vi "Normalize Results.vi"(8 "Sorted Data":dbl[][](array[numeric]), 11 "Image in":T2) -> (3 "Results":T1(array[cluster]) {"Score" format="%#_3g"; "Pixels"."Rectangle"."Numeric 5" format="%#_3g"; "Pixels"."Rectangle"."Numeric 3" format="%#_3g"; "Pixels"."Rectangle"."Numeric 2" format="%#_3g"; "Pixels"."Rectangle"."Numeric" format="%#_3g"; "Normalized"."Rectangle"."Numeric 5" format="%#_2g"; "Normalized"."Rectangle"."Numeric 3" format="%#_2g"; "Normalized"."Rectangle"."Numeric 2" format="%#_2g"; "Normalized"."Rectangle"."Numeric" format="%#_2g"; "Normalized"."Center"."?" format="%#_3g"; "Normalized"."Center"."?" format="%#_3g"; "Distance (ft)" format="%#_3g"})   [LabVIEW 2016]
uses:
  <vilib>/vision/Image Controls.llb/IMAQ Image.ctl
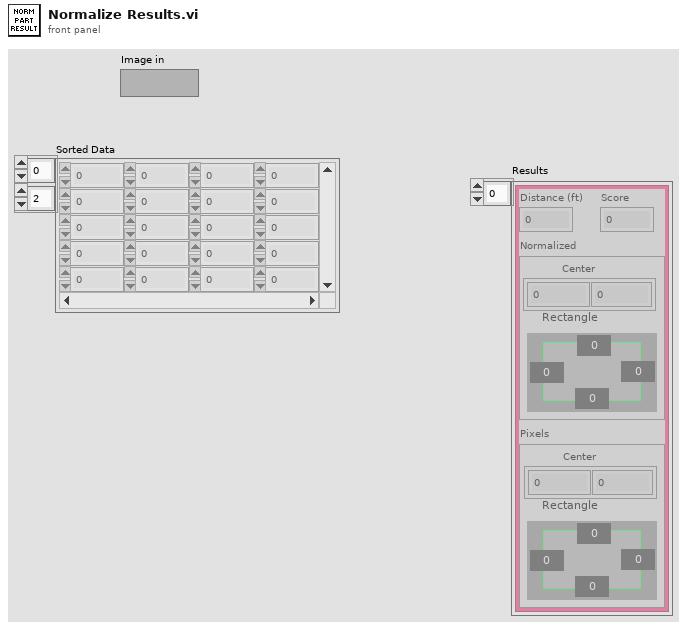
[diagram p1: front panel]
types:
  T1 = cluster{"Distance (ft)":dbl, "Score":dbl, "Normalized":cluster{"Center":cluster{dbl, dbl}, "Rectangle":cluster{"Numeric":dbl, "Numeric 2":dbl, "Numeric 3":dbl, "Numeric 5":dbl}}, "Pixels":cluster{"Center":cluster{dbl, dbl}, "Rectangle":cluster{"Numeric":dbl, "Numeric 2":dbl, "Numeric 3":dbl, "Numeric 5":dbl}}}[]
  T2 = typedef "IMAQ Image.ctl" = refnum<image>
  T3 = cluster{"left":dbl, "top":dbl, "right":dbl, "bottom":dbl}
  T4 = cluster{"Distance (ft)":dbl, "Score":dbl, "Normalized":cluster{"Center":cluster{dbl, dbl}, "Rectangle":cluster{"Numeric":dbl, "Numeric 2":dbl, "Numeric 3":dbl, "Numeric 5":dbl}}, "Pixels":cluster{"Center":cluster{dbl, dbl}, "Rectangle":cluster{"Numeric":dbl, "Numeric 2":dbl, "Numeric 3":dbl, "Numeric 5":dbl}}}
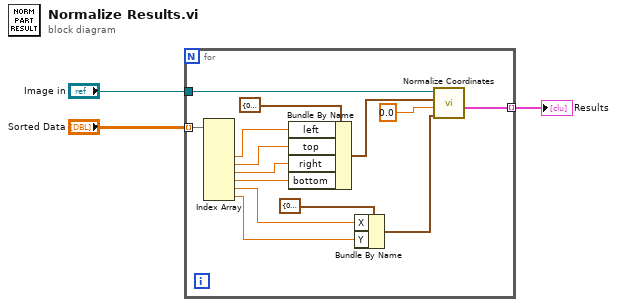
[diagram p0: block diagram]
diagram:
  n1 = for {
    tunnel: "Image in" -> [w17]
    tunnel: "Sorted Data" -> [w15] mode=indexing
    tunnel: [w4] -> w1 mode=indexing
    n2 = Index Array(array=w15) -> (element #3=w14:dbl, element #4=w13:dbl, element #5=w12:dbl, element #6=w11:dbl, element #7=w6:dbl, element #8=w5:dbl)  [unwired: 8 in, 2 out]
    n3 = Bundle By Name(cluster=T3 {"left"=0.0, "top"=0.0, "right"=0.0, "bottom"=0.0} ("Bounding box"), "left"=w14, "top"=w13, "right"=w12, "bottom"=w11) -> (w10:T3)
    n4 = Bundle By Name(cluster=cluster{"X":dbl, "Y":dbl} {"X"=0.0, "Y"=0.0} ("Center"), "X"=w6, "Y"=w5) -> (w7:cluster{"X":dbl, "Y":dbl})
    n5 = call "Normalize Coordinates.vi"("Center"=w7, "Distance"=0.0, "Bounding box"=w10, "Image in"=w17) -> ("Results"=w4:T4)  [unwired: 6 in, 1 out]
  }
  "Results" <- w1
